vi "_DServerSetClassTimeoutInSec.vi"(3 "error in":errorcluster, 4 "client request timeout in sec":dbl=3.0, 5 "class name":string="unspecified_device_name") -> (0 "error out":errorcluster)   [LabVIEW 2014, in "tango.lvlib"]
uses:
  tango.lvlib
  tango_binding.so
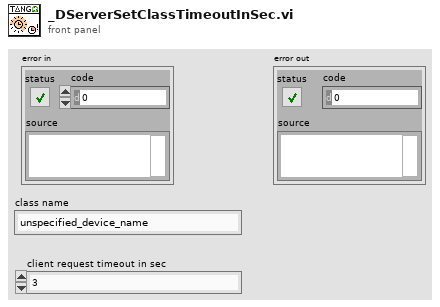
[diagram p1: front panel]
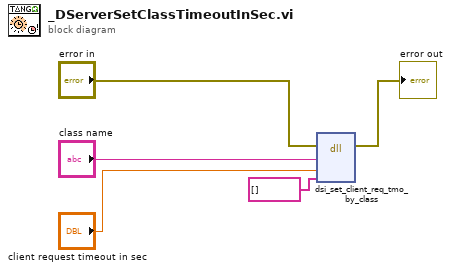
[diagram p0: block diagram]
diagram:
  n1 = dll-call lib="tango_binding.*" fn="dsi_set_client_req_tmo_by_class"(error in="error in", "device_name"="class name", "timeout_in_sec"="client request timeout in sec", "error_stack"=string[] [] ("error stack")) -> (error out=→"error out":errorcluster)  [unwired: 6 in, 1 out]
